vi "v2 clear all errors.vi"(11 "h":u32) -> (2 "function return":i32, 3 "h out":u32)   [LabVIEW 2019, in "apdm.lvlib"]
doc: "APDM_EXPORT int apdm_v2_clear_all_errors(apdm_device_handle_t h);"
uses:
  apdm.lvlib
  Lee Lab/CP FES Walking 2018/Code/Working/LabVIEW/apdm.dll
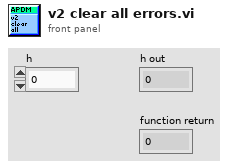
[diagram p1: front panel]
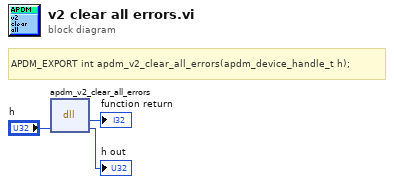
[diagram p0: block diagram]
diagram:
  # "APDM_EXPORT int apdm_v2_clear_all_errors(apdm_device_handle_t h);"
  n1 = dll-call lib="C:/Users/jfalesi/Dropbox/Lee Lab/CP FES Walking 2018/Code/Working/LabVIEW/apdm.*" fn="apdm_v2_clear_all_errors"("h"="h") -> (→"function return":i32, "h"=→"h out":u32)  [unwired: 3 in, 2 out]
